vi "CalcBallVel.vi"(4 "initialize":bool, 10 "fps":dbl, 11 "balls":T1[](array[typedef])) -> (3 "balls out":T1[](array[typedef]))   [LabVIEW 2023, in "Vision.lvclass"]
uses:
  Vision.lvclass
  <vilib>/Analysis/Matrix/Datatypes/RealMatrix.ctl
  <vilib>/Analysis/Matrix/NI_Matrix.lvlib
  Old vision/Controls/SSL Detection Ball.ctl
  Utilities_class/Utilities.lvclass
  <vilib>/ptbypt/NI_PtbyPt.lvlib
  <vilib>/Analysis/3filter.llb/Filter Passband Type.ctl
  <vilib>/Analysis/NI_AALBase.lvlib
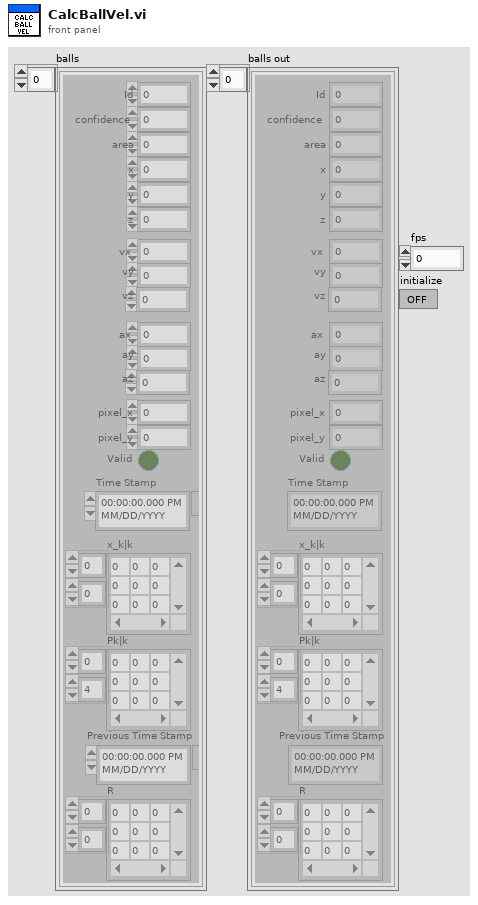
[diagram p1: front panel]
types:
  T1 = typedef "SSL Detection Ball.ctl" = cluster{"x":sgl, "area":u32, "confidence":sgl, "y":sgl, "z":sgl, "pixel_x":sgl, "pixel_y":sgl, "Valid":bool, "Time Stamp":timestamp, "x_k|k":T2, "Pk|k":T2, "Id":u32, "Previous Time Stamp":timestamp, "R":T2, " vx":sgl, "vy":dbl, "vz":dbl, " ax":sgl, "ay":dbl, "az":dbl}
  T2 = typedef "NI_Matrix.lvlib/RealMatrix.ctl" = dbl[][]
  T3 = typedef "NI_AALBase.lvlib/Filter Passband Type.ctl" = enum32{"Lowpass", "Highpass", "Bandpass", "Bandstop"}
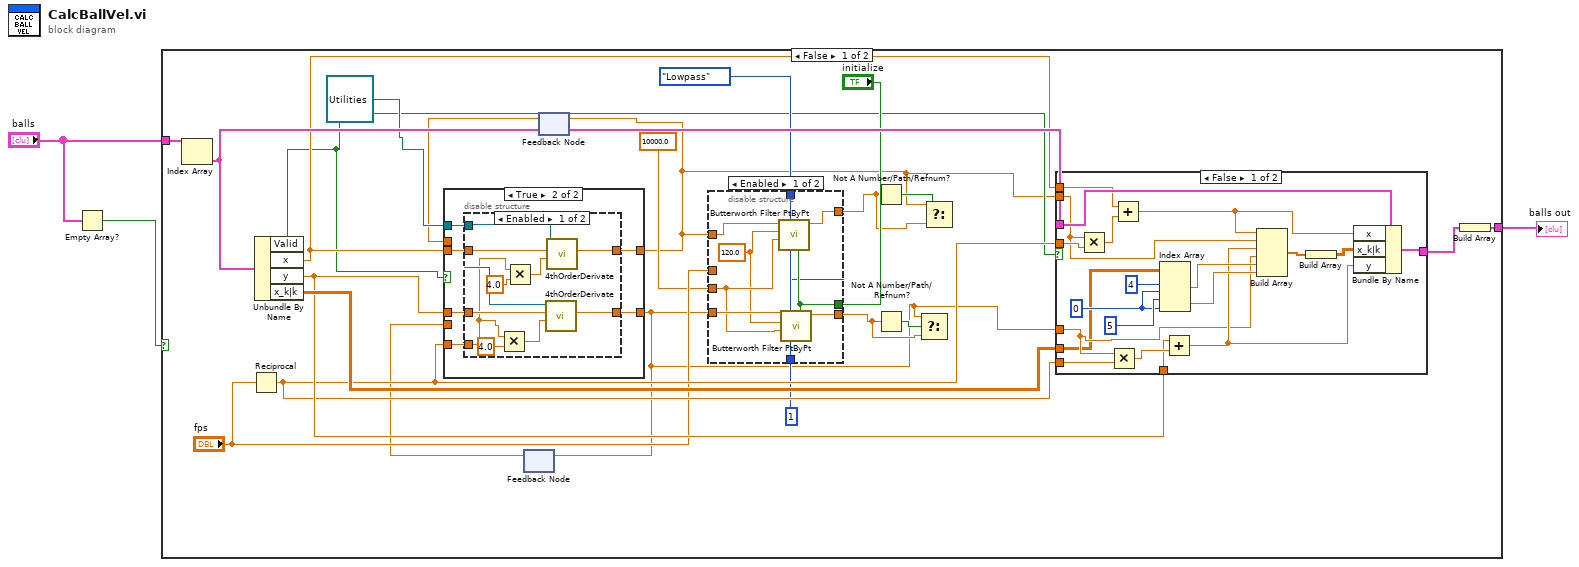
[diagram p0: block diagram]
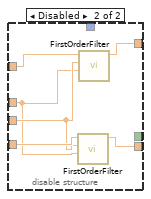
[diagram p2: hidden frame]
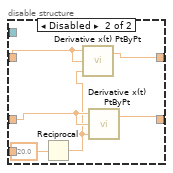
[diagram p4: hidden frame]
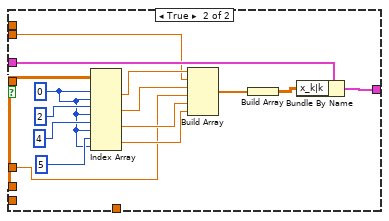
[diagram p5: hidden frame]
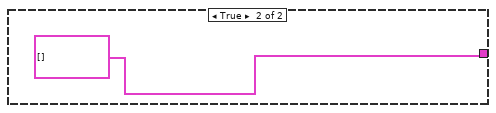
[diagram p6: hidden frame]
diagram:
  n1 = Empty Array?(array="balls") -> (empty?=w1:bool)
  n2 = case shown="False" w1 {
    tunnel: [w25 T1[] []] -> w3
    tunnel: "balls" -> [w22 _]
    frame False {
      n3 = Index Array(array=w22) -> (element=w26:T1)  [unwired: 1 in]
      n4 = Reciprocal(x="fps") -> (1/x=w18:dbl)
      n5 = Unbundle By Name(w26) -> ("Valid"=w8:bool, "x"=w21:sgl, "y"=w20:sgl, "x_k|k"=w23:T2)
      n6 = feedback #1() -> (w6:dbl)  [unwired: 1 in]
      n7 = feedback #2() -> (w7:dbl)  [unwired: 1 in]
      n8 = case shown="True" w8 {
        tunnel: w21 -> [_ w49]
        tunnel: w20 -> [_ w48]
        tunnel: refnum<class "Utilities.lvclass"> refnum ("Utilities in") -> [_ w47]
        tunnel: w18 -> [_ w46]
        tunnel: [w43 w45] -> w5
        tunnel: [w42 w44] -> w4
        tunnel: w7 -> [w43 _]
        tunnel: w6 -> [w42 _]
        frame False {
        }
        frame True {
          n9 = disable-structure shown="Enabled" {
            disable-tunnel: w49 -> [w59 w65]
            disable-tunnel: w48 -> [w58 w64]
            disable-tunnel: w47 -> [w57 _]
            disable-tunnel: w46 -> [w54 _]
            disable-tunnel: [w56 w60] -> w45
            disable-tunnel: [w55 w61] -> w44
            frame Enabled {
              n10 = Multiply(x=w54, y=4.0) -> (x*y=w50:dbl)
              n11 = Multiply(x=w54, y=4.0) -> (x*y=w51:dbl)
              n12 = call "4thOrderDerivate.vi"("dt"=w50, "x"=w58, "Utilities in"=w57) -> ("dx/dt"=w55:dbl)  [unwired: 6 in, 2 out]
              n13 = call "4thOrderDerivate.vi"("dt"=w51, "x"=w59, "Utilities in"=w57) -> ("dx/dt"=w56:dbl)  [unwired: 6 in, 2 out]
            }
            frame Disabled {
              n14 = Reciprocal(x=120.0) -> (1/x=w62:dbl)
              n15 = call <vilib>:"Derivative x(t) PtByPt.vi"("dt"=w62, "initial condition"=w65, "x"=w65) -> ("dx/dt"=w60:dbl)  [unwired: 1 in, 1 out]
              n16 = call <vilib>:"Derivative x(t) PtByPt.vi"("dt"=w62, "initial condition"=w64, "x"=w64) -> ("dx/dt"=w61:dbl)  [unwired: 1 in, 1 out]
            }
          }
        }
      }
      n17 = feedback-in #1(w4) -> ()
      n18 = feedback-in #2(w5) -> ()
      n19 = disable-structure shown="Enabled" {
        disable-tunnel: "fps" -> [_ w38]
        disable-tunnel: 10000.0 -> [w28 w39]
        disable-tunnel: 1 ("order") -> [w35 _]
        disable-tunnel: "initialize" -> [w34 _]
        disable-tunnel: Filter_Passband_Type."Lowpass" ("filter type") -> [w33 _]
        disable-tunnel: [w32 w37] -> w11
        disable-tunnel: [w31 w36] -> w9
        disable-tunnel: w5 -> [w29 w40]
        disable-tunnel: w4 -> [w30 w41]
        frame Enabled {
          w27 = 120.0
          n20 = call <vilib>:"Butterworth Filter PtByPt.vi"("initialize"=w34, "order"=w35, "filter type"=w33, "high cutoff freq: fh"=w28, "sampling freq: fs"=w27, "x"=w29) -> ("Filtered x"=w32:dbl)  [unwired: 3 in, 1 out]
          n21 = call <vilib>:"Butterworth Filter PtByPt.vi"("initialize"=w34, "order"=w35, "filter type"=w33, "high cutoff freq: fh"=w28, "sampling freq: fs"=w27, "x"=w30) -> ("Filtered x"=w31:dbl)  [unwired: 3 in, 1 out]
        }
        frame Disabled {
          n22 = call "FirstOrderFilter.vi"("fps"=w38, "fc"=w39, "Numeric in"=w41) -> ("Numeric out"=w36:dbl)  [unwired: 8 in]
          n23 = call "FirstOrderFilter.vi"("fps"=w38, "fc"=w39, "Numeric in"=w40) -> ("Numeric out"=w37:dbl)  [unwired: 8 in]
        }
      }
      n24 = Not A Number/Path/Refnum?(number/path/refnum=w11) -> (NaN/Path/Refnum?=w13:bool)
      n25 = Not A Number/Path/Refnum?(number/path/refnum=w9) -> (NaN/Path/Refnum?=w10:bool)
      n26 = Select(t=w4, s=w10, f=w9) -> ()  [unwired: 1 out]
      n27 = Select(t=w5, s=w13, f=w11) -> ()  [unwired: 1 out]
      n28 = case shown="False" w8 {
        tunnel: w26 -> [w82 w100]
        tunnel: [w72 w99] -> w24
        tunnel: w23 -> [w67 w87]
        tunnel: w5 -> [w69 w90]
        tunnel: w4 -> [w68 w89]
        tunnel: w18 -> [w77 _]
        tunnel: w18 -> [w76 _]
        tunnel: w21 -> [w74 _]
        tunnel: w20 -> [w73 _]
        frame False {
          w81 = 0
          n29 = Multiply(x=w69, y=w77) -> (x*y=w78:dbl)
          n30 = Multiply(x=w68, y=w76) -> (x*y=w75:dbl)
          n31 = Add(x=w74, y=w78) -> (x+y=w71:dbl)
          n32 = Index Array(array=w67, index (row) #1=4, index (col) #1=w81, index (row) #2=5, index (col) #2=w81) -> (element #1=w80:dbl, element #2=w79:dbl)
          n33 = Add(x=w73, y=w75) -> (x+y=w70:dbl)
          n34 = Build Array(w71, w69, w70, w68, w80, w79) -> (w85:dbl[])
          n35 = Build Array(w85) -> (w66:T2)
          n36 = Bundle By Name(cluster=w82, "x"=w71, "x_k|k"=w66, "y"=w70) -> (w72:T1)
        }
        frame True {
          w88 = 0
          n37 = Index Array(array=w87, index (row) #1=w88, index (col) #1=w88, index (row) #2=2, index (col) #2=w88, index (row) #3=4, index (col) #3=w88, index (row) #4=5, index (col) #4=w88) -> (element #1=w94:dbl, element #2=w93:dbl, element #3=w92:dbl, element #4=w91:dbl)
          n38 = Build Array(w94, w90, w93, w89, w92, w91) -> (w98:dbl[])
          n39 = Build Array(w98) -> (w86:T2)
          n40 = Bundle By Name(cluster=w100, "x_k|k"=w86) -> (w99:T1)
        }
      }
      n41 = Build Array(w24) -> (w25:T1[])
    }
    frame True {
    }
  }
  "balls out" <- w3
